vi "Introspection Core.vi"(8 "error in (no error)":errorcluster, 11 "IVI_Fgen in":refnum<class "IVI_Fgen.lvclass">) -> (0 "error out":errorcluster, 2 "CS++Messages":refnum<class "Message.lvclass">[](array[class]), 3 "IVI_Fgen out":refnum<class "IVI_Fgen.lvclass">)   [LabVIEW 2014, in "IVI_Fgen.lvlib" / "IVI_Fgen.lvclass"]
doc: "This vi delivers a list with all messages this actor reacts to. \n\nNote that all inherited classes have to overwrite it."
uses:
  IVI_Fgen.lvclass
  <vilib>/ActorFramework/Message/Message.lvclass
  CSPP_DeviceBase/CS++Fgen/CS++Fgen.lvclass
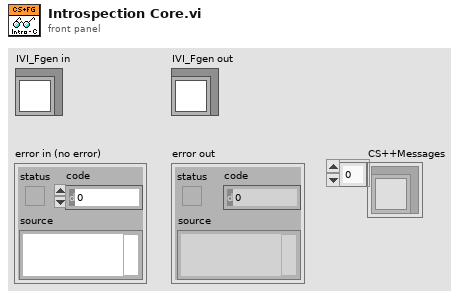
[diagram p1: front panel]
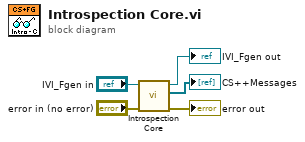
[diagram p0: block diagram]
diagram:
  n1 = call-parent "Introspection Core.vi"("error in (no error)"="error in (no error)", "CS++Fgen in"="IVI_Fgen in") -> ("error out"=→"error out":errorcluster, "CS++Messages"=→"CS++Messages":refnum<class "Message.lvclass">[], "CS++Fgen out"=→"IVI_Fgen out":refnum<class "IVI_Fgen.lvclass">)  [unwired: 7 in]
